vi "CmdexBuzzer.vi"(0 "Error Input":errorcluster, 5 "interval":u16=100, 7 "frequency":u16=500, 9 "power":u16=80, 11 "Uart Input":cluster{u64} {"?" format="%x"}) -> (4 "Error Output":errorcluster, 15 "Uart Output":cluster{u64} {"?" format="%x"})   [LabVIEW 2019]
doc: "<B>Cmdex</B>\nBeep sound."
uses:
  dll/LabViewUart.dll
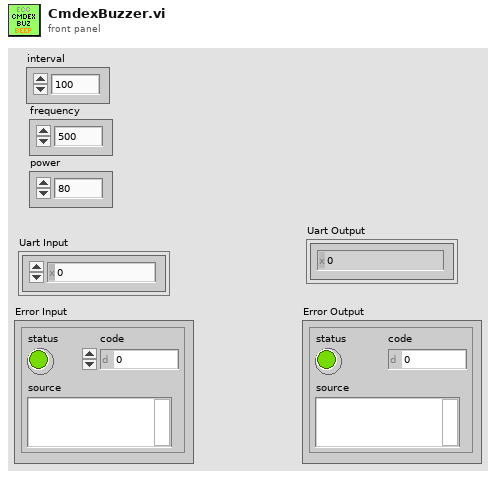
[diagram p1: front panel]
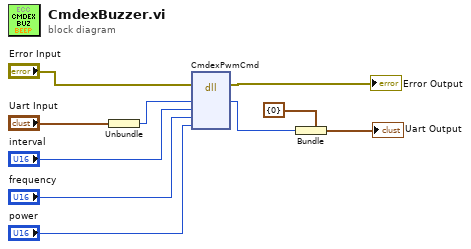
[diagram p0: block diagram]
diagram:
  n1 = Unbundle("Uart Input") -> (w7:u64)
  n2 = dll-call lib="D:/Google Drive/INC-2020/INC352/INC352-2020/LabVIEW/examples/uart-cmdex/SubVI/dll/LabViewUart.dll" fn="CmdexPwmCmd"(error in="Error Input", "Uart Handle"=w7, "interval"="interval", "frequency"="frequency", "power"="power") -> (error out=→"Error Output":errorcluster, "Uart Handle"=w4:u64)  [unwired: 6 in, 1 out]
  n3 = Bundle(cluster=cluster{u64} {0}, w4) -> (→"Uart Output":cluster{u64})
